vi "Trapezoidal Motion Profile.vi"(7 "Reset?":bool, 10 "Distance":dbl) -> (2 "Throttle Out":sgl, 4 "Finished?":bool)   [LabVIEW 2015]
uses:
  Robot Code/Robot Global Data.vi
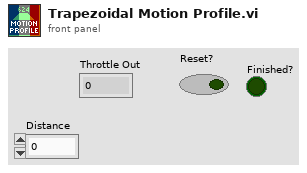
[diagram p1: front panel]
types:
  T1 = typedef "Dashboard Control Data.ctl" = cluster{"Shooter Presets":T2, "Encoder Control":T4, "Steer PID output":cluster{"output high":dbl, "output low":dbl}, " Steer PID gains":cluster{"proportional gain (Kc)":dbl, "integral time (Ti, min)":dbl, "derivative time (Td, min)":dbl}, "Drivetrain Settings":T5, "Vision Packet":T6, "Dashboard Drivetrain Command":T7, "Info/Command Cluster":T9, "Ball Vision Packet":T10, "Intake Presets":T12, "Intake Encoder Control":T14, "Climb Presets":T15, "Ultrasonic Limit":dbl, "Roll Limit":dbl, "Pitch Limit":dbl, "Goal Output Range":cluster{"output high":dbl, "output low":dbl}}
  T2 = typedef "Shooter Presets.ctl" = cluster{"Batter Shot":T3, "Deep Middle Shot":T3, "Manual Shot":T3, "Left Ticks Per Rotation":dbl, "Right Ticks Per Rotation":dbl, "Low Bar Shot":T3, "Shooter RPM Tolerance":dbl, "IIR Filter Power":dbl, "Trigger Power":dbl, "Fire from Load Delay":i32, "Angle Pot M":dbl, "Angle Pot B":dbl, "Shooter Length":dbl, "String Pot Dist":dbl, "Angle PID gains":cluster{"proportional gain (Kc)":dbl, "integral time (Ti, min)":dbl, "derivative time (Td, min)":dbl}, "Angle Motor Output":cluster{"output high":dbl, "output low":dbl}, "Shooter Angle Tolerance":dbl, "Vision Shoot x^2":dbl, "Vision Shoot x":dbl, "Dist from Axis Cam to Pivot":dbl, "High Goal Center Height":dbl, "Feed Forward Max Accel":dbl, "Feed Forward Kv":dbl, "Backwards Trigger":dbl, "Shot Finish Delay (ms)":dbl, "Angle Max Current":dbl, "Angle Current Trip Time":dbl, "Shooter Intake Angle":dbl, "Vision Shoot c":dbl, "Reset?":bool, "Servo Release Delay":dbl, "Servo Idle Angle":i32, "Servo Hold Angle":i32, "Angle Pot x^2":dbl, "Angle Pot x":dbl, "Angle Pot c":dbl, "Ignore Angle?":bool}
  T3 = typedef "Shot Presets.ctl" = cluster{"Left Wheel RPM":dbl, "Right Wheel RPM":dbl, "Angle":dbl}
  T4 = typedef "Encoder Control.ctl" = cluster{"Right Tick Constant":dbl, "Left Tick Constant":dbl, "Reset?":bool, "Y Dist":cluster{"PID gains":cluster{"proportional gain (Kc)":dbl, "integral time (Ti, min)":dbl, "derivative time (Td, min)":dbl}}, "Y Stop Thresh":dbl, "Y Stop Speed":dbl}
  T5 = typedef "Drivetrain Settings.ctl" = cluster{"Gyro Tolerance":dbl, "Throttle Ramp (ms)":dbl, "Angular rate compensation":bool, "Throttle to Rate Scale":dbl, "Rate compensation gain":dbl, "Kv":dbl, "Ka":dbl, "Feed Forward P":dbl, "Feed Forward D":dbl, "Goal Vision PID gains":cluster{"proportional gain (Kc)":dbl, "integral time (Ti, min)":dbl, "derivative time (Td, min)":dbl}, "Goal Detection Window":dbl}
  T6 = typedef "Goal Vision Packet.ctl" = cluster{"Distance":dbl, "Center X":dbl, "Center Y":dbl, "Found Target?":bool}
  T7 = typedef "Dashboard Drivetrain Command.ctl" = cluster{"Drivetrain Vision":T8}
  T8 = typedef "Drivetrain Vision.ctl" = cluster{"Goal Window":dbl, "Ball Window":dbl}
  T9 = typedef "Ball Tracking Command Cluster.ctl" = cluster{"Distance to Ball":dbl, "Desired Angle":dbl, "Command":enum16{"Turn to Ball", "Turn to Angle", "Get Distance"}, "Pixels from Center":dbl}
  T10 = typedef "Ball Vision Packet.ctl" = cluster{"Ball Detected?":bool, "Distance to Ball":dbl, "Desired Angle":dbl, "Pixels from Center":dbl, "Tracking mode":T11}
  T11 = typedef "Tracking Mode.ctl" = enum16{"Turn to Ball", "Turn to Angle"}
  T12 = typedef "Intake Presets.ctl" = cluster{"Intake Speed":dbl, "Outake Speed":dbl, "Low Height":dbl, "Half Height":dbl, "Full Height":dbl, "Angle Speed":dbl, "Fast Angle":dbl, "Encoder Scale":dbl, "Load Height":dbl, "Output Range":T13, "Rotation Power Max/Min":dbl, "MaxCurrent":dbl, "Intake Trip Time":dbl, "Idle Height":dbl, "Max Height":dbl, "Reset Encoders?":bool, "PID gains":cluster{"proportional gain (Kc)":dbl, "integral time (Ti, min)":dbl, "derivative time (Td, min)":dbl}}
  T13 = typedef "Drivetrain Output Range.ctl" = cluster{"output high":dbl, "output low":dbl}
  T14 = typedef "IntakeEcoderControl.ctl" = cluster{"Arm Tick Constant":dbl, "Reset?":bool, "Y Dist":cluster{"PID gains":cluster{"proportional gain (Kc)":dbl, "integral time (Ti, min)":dbl, "derivative time (Td, min)":dbl}}, "Y Stop Thresh":dbl, "Y Stop Speed":dbl}
  T15 = typedef "Climb Presets.ctl" = cluster{"Pull Power":dbl, "Unpin Power":dbl, "Time to Hold":dbl}
  T16 = typedef "Encoder Values Super Cluster.ctl" = cluster{"Left Encoder":T17, "Right Encoder":T17}
  T17 = typedef "Encoder Values.ctl" = cluster{"Distance":dbl, "Speed":dbl, "Ticks":dbl}
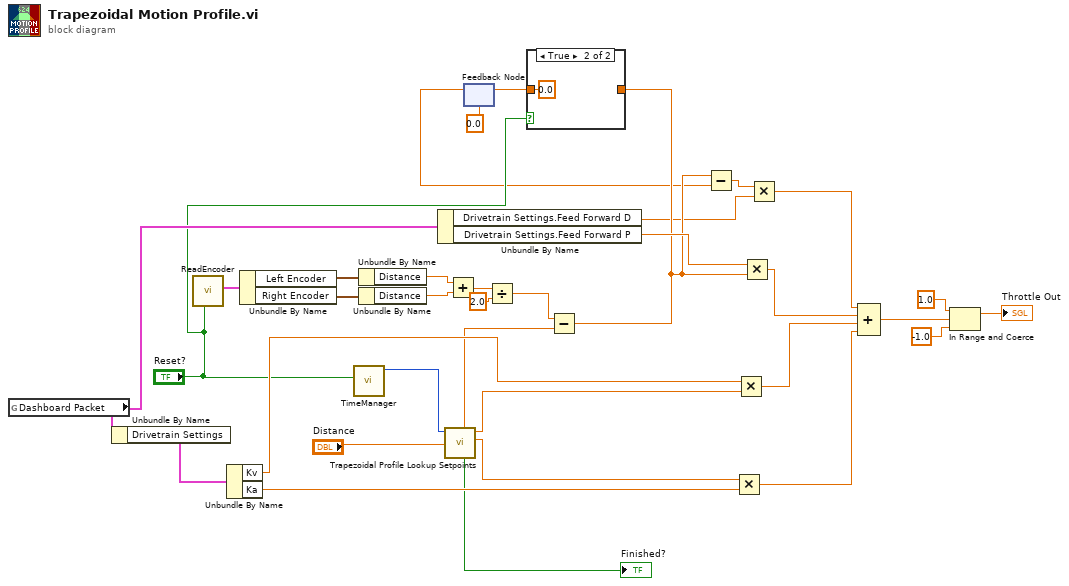
[diagram p0: block diagram]
diagram:
  n1 = global read "Robot Global Data.vi" "Dashboard Packet"() -> (w14:T1)
  n2 = Unbundle By Name(w14) -> ("Drivetrain Settings"=w27:T5)
  n3 = call "ReadEncoder.vi"("Reset?"="Reset?") -> ("Quick Use Cluster"=w24:T16)  [unwired: 10 in]
  n4 = Unbundle By Name(w27) -> ("Kv"=w26:dbl, "Ka"=w25:dbl)
  n5 = Unbundle By Name(w24) -> ("Left Encoder"=w23:T17, "Right Encoder"=w22:T17)
  n6 = call "TimeManager.vi"("Reset?"="Reset?") -> ("Time Since Reset"=w34:u32)  [unwired: 9 in, 1 out]
  n7 = Unbundle By Name(w23) -> ("Distance"=w21:dbl)
  n8 = Unbundle By Name(w22) -> ("Distance"=w20:dbl)
  n9 = Unbundle By Name(w14) -> ("Drivetrain Settings.Feed Forward D"=w6:dbl, "Drivetrain Settings.Feed Forward P"=w13:dbl)
  n10 = call "Trapezoidal Profile Lookup Setpoints.vi"("Total Distance"="Distance", "Current Time"=w34) -> ("Acceleration"=w30:sgl, "Velocity"=w29:sgl, "Profile Completed?"=→"Finished?":bool, "Projected Current Distance"=w16:dbl)  [unwired: 6 in]
  n11 = Add(x=w21, y=w20) -> (x+y=w19:dbl)
  n12 = feedback #1(0.0) -> (w8:dbl)
  n13 = Divide(x=w19, y=2.0) -> (x/y=w15:dbl)
  n14 = Subtract(x=w15, y=w16) -> (x-y=w9:dbl)
  n15 = case shown="True" "Reset?" {
    tunnel: [w35 0.0] -> w11
    tunnel: w9 -> [w35 _]
    frame False {
    }
    frame True {
    }
  }
  n16 = feedback-in #1(w11) -> ()
  n17 = Subtract(x=w9, y=w8) -> (x-y=w7:dbl)
  n18 = Multiply(x=w30, y=w25) -> (x*y=w2:dbl)
  n19 = Multiply(x=w26, y=w29) -> (x*y=w3:dbl)
  n20 = Multiply(x=w13, y=w9) -> (x*y=w4:dbl)
  n21 = Multiply(x=w7, y=w6) -> (x*y=w5:dbl)
  n22 = Compound Arithmetic op=ADD(w5, w4, w3, w2) -> (w1:dbl)
  n23 = In Range and Coerce(upper limit=sgl 1.0, x=w1, lower limit=sgl -1.0) -> (coerced(x)=→"Throttle Out":dbl)  [unwired: 1 out]
